vi "流程写入.vi"(11 "添加的路径":path) -> ()   [LabVIEW 2016, in "斯坦道总磷.lvlib"]
uses:
  <vilib>/Utility/miscctls.llb/LVPointTypeDef.ctl
panel:
  in  "关闭":bool
  out "字符串":string
  in  "加标回收":bool
  in  "标样核查":bool
  in  "跨度核查":bool
  in  "零点核查":bool
  in  "水样测量":bool=TRUE
  in  "写入":bool
  in  "参数下拉列表":enum16{"总磷", "总氮", "氨氮"}(ring)
  in  "量程下拉列表":enum16{"低量程", "高量程"}(ring)
  # "请选择要写入的流程"
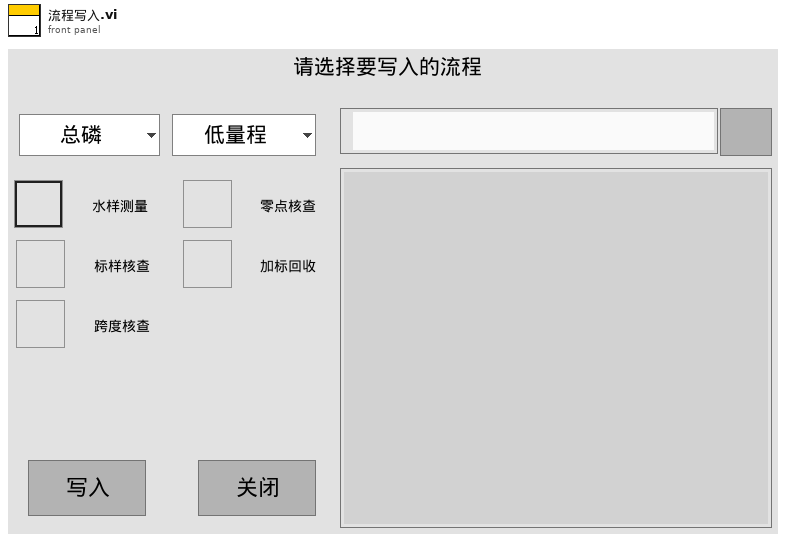
[diagram p1: front panel]
types:
  T1 = typedef "LVPointTypeDef.ctl" = cluster{"Horizontal":i16, "Vertical":i16}
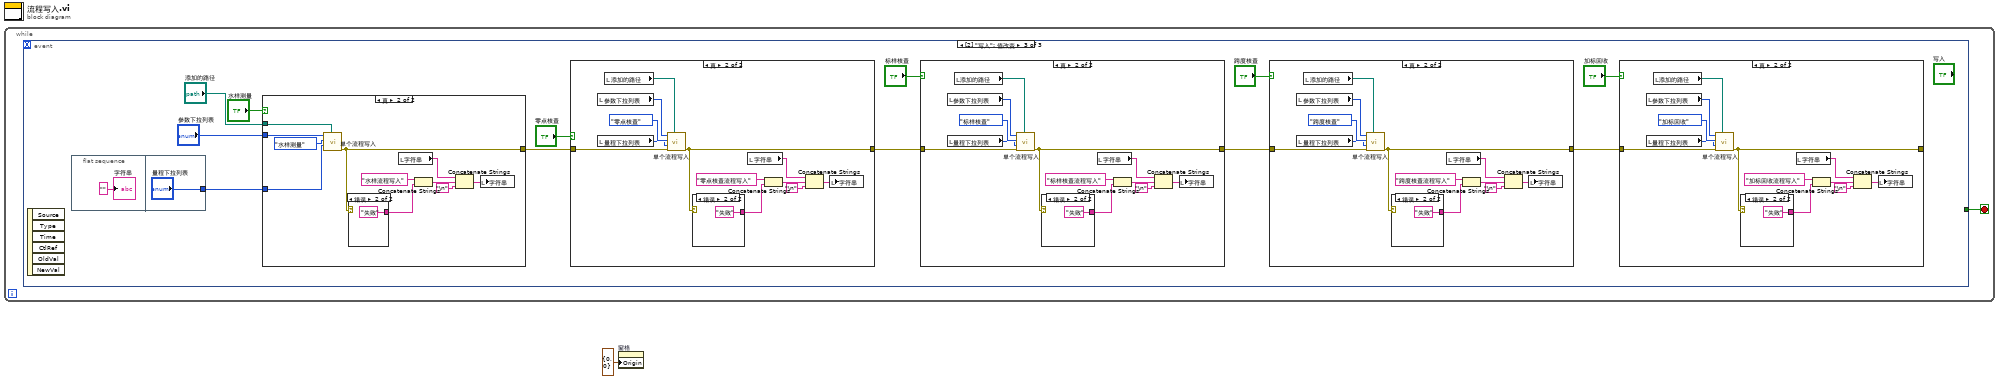
[diagram p0: block diagram]
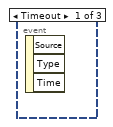
[diagram p2: hidden frame]
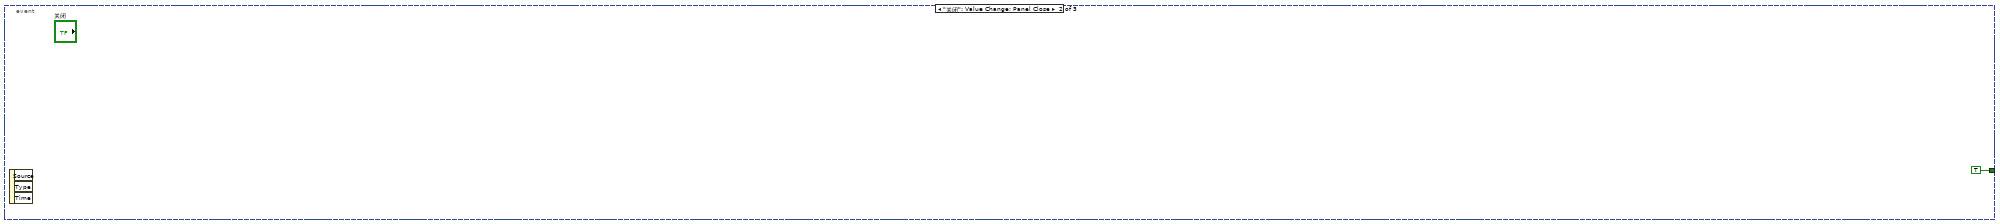
[diagram p3: hidden frame]
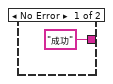
[diagram p5: hidden frame]
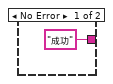
[diagram p7: hidden frame]
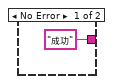
[diagram p9: hidden frame]
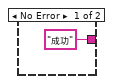
[diagram p11: hidden frame]
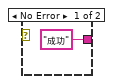
[diagram p13: hidden frame]
diagram:
  n1 = while {
    stop <- w2 stop-if-true
    n2 = event shown="[2] \"写入\": 值改变" {
      selector: _ -> [_ _ _]
      dyn-events: _ -> [_ _ _]
      timeout: _ -> [_ _ _]
      tunnel: [_ TRUE _] -> w2
      event Timeout {
        n3 = event-data() -> ()  [unwired: 1 in, 3 out]
      }
      event "关闭": Value Change; Panel Close {
        n4 = event-data() -> ()  [unwired: 1 in, 3 out]
      }
      event "写入": Value Change {
        n5 = event-data() -> ()  [unwired: 1 in, 6 out]
        n6 = flat-sequence {
          tunnel: ["量程下拉列表"] -> w14
          frame #0 {
            "字符串" <- ""
          }
          frame #1 {
          }
        }
        n7 = case shown="真" "水样测量" {
          tunnel: "添加的路径" -> [_ w84]
          tunnel: "参数下拉列表" -> [_ w83]
          tunnel: w14 -> [_ w82]
          tunnel: [_ w80] -> w11
          frame False {
          }
          frame True {
            n8 = call "单个流程写入.vi"("添加的路径"=w84, "量程"=w82, "测量模式"=enum16{"水样测量", "零点核查", "跨度核查", "标样核查", "加标回收"}."水样测量", "测量参数"=w83) -> ("error out"=w80:errorcluster)  [unwired: 7 in]
            n9 = case shown="错误" w80 {
              tunnel: ["成功" "失败"] -> w77
              frame No Error {
              }
              frame Error {
              }
            }
            n10 = local read "字符串"() -> (w79:string)
            n11 = Concatenate Strings("水样流程写入", w77) -> (w76:string)
            n12 = Concatenate Strings(w79, w76, "\n") -> (w74:string)
            n13 = local write "字符串"(w74) -> ()
          }
        }
        n14 = case shown="真" "零点核查" {
          tunnel: [_ w70] -> w9
          tunnel: w11 -> [_ w60]
          frame False {
          }
          frame True {
            n15 = local read "参数下拉列表"() -> (w62:enum16{"总磷", "总氮", "氨氮"})
            n16 = local read "量程下拉列表"() -> (w61:enum16{"低量程", "高量程"})
            n17 = local read "添加的路径"() -> (w63:path)
            n18 = call "单个流程写入.vi"("添加的路径"=w63, "error in (no error)"=w60, "量程"=w61, "测量模式"=enum16{"水样测量", "零点核查", "跨度核查", "标样核查", "加标回收"}."零点核查", "测量参数"=w62) -> ("error out"=w70:errorcluster)  [unwired: 6 in]
            n19 = case shown="错误" w70 {
              tunnel: ["成功" "失败"] -> w67
              frame No Error {
              }
              frame Error {
              }
            }
            n20 = local read "字符串"() -> (w69:string)
            n21 = Concatenate Strings("零点核查流程写入", w67) -> (w66:string)
            n22 = Concatenate Strings(w69, w66, "\n") -> (w64:string)
            n23 = local write "字符串"(w64) -> ()
          }
        }
        n24 = case shown="真" "标样核查" {
          tunnel: [_ w56] -> w7
          tunnel: w9 -> [_ w46]
          frame False {
          }
          frame True {
            n25 = local read "参数下拉列表"() -> (w48:enum16{"总磷", "总氮", "氨氮"})
            n26 = local read "量程下拉列表"() -> (w47:enum16{"低量程", "高量程"})
            n27 = local read "添加的路径"() -> (w49:path)
            n28 = call "单个流程写入.vi"("添加的路径"=w49, "error in (no error)"=w46, "量程"=w47, "测量模式"=enum16{"水样测量", "零点核查", "跨度核查", "标样核查", "加标回收"}."标样核查", "测量参数"=w48) -> ("error out"=w56:errorcluster)  [unwired: 6 in]
            n29 = case shown="错误" w56 {
              tunnel: ["成功" "失败"] -> w53
              frame No Error {
              }
              frame Error {
              }
            }
            n30 = local read "字符串"() -> (w55:string)
            n31 = Concatenate Strings("标样核查流程写入", w53) -> (w52:string)
            n32 = Concatenate Strings(w55, w52, "\n") -> (w50:string)
            n33 = local write "字符串"(w50) -> ()
          }
        }
        n34 = case shown="真" "跨度核查" {
          tunnel: [_ w32] -> w4
          tunnel: w7 -> [_ w33]
          frame False {
          }
          frame True {
            n35 = local read "参数下拉列表"() -> (w35:enum16{"总磷", "总氮", "氨氮"})
            n36 = local read "量程下拉列表"() -> (w34:enum16{"低量程", "高量程"})
            n37 = local read "添加的路径"() -> (w36:path)
            n38 = call "单个流程写入.vi"("添加的路径"=w36, "error in (no error)"=w33, "量程"=w34, "测量模式"=enum16{"水样测量", "零点核查", "跨度核查", "标样核查", "加标回收"}."跨度核查", "测量参数"=w35) -> ("error out"=w32:errorcluster)  [unwired: 6 in]
            n39 = case shown="错误" w32 {
              tunnel: ["成功" "失败"] -> w40
              frame No Error {
              }
              frame Error {
              }
            }
            n40 = local read "字符串"() -> (w42:string)
            n41 = Concatenate Strings("跨度核查流程写入", w40) -> (w39:string)
            n42 = Concatenate Strings(w42, w39, "\n") -> (w37:string)
            n43 = local write "字符串"(w37) -> ()
          }
        }
        n44 = case shown="真" "加标回收" {
          tunnel: [_ w28] -> _
          tunnel: w4 -> [_ w18]
          frame False {
          }
          frame True {
            n45 = local read "参数下拉列表"() -> (w20:enum16{"总磷", "总氮", "氨氮"})
            n46 = local read "量程下拉列表"() -> (w19:enum16{"低量程", "高量程"})
            n47 = local read "添加的路径"() -> (w21:path)
            n48 = call "单个流程写入.vi"("添加的路径"=w21, "error in (no error)"=w18, "量程"=w19, "测量模式"=enum16{"水样测量", "零点核查", "跨度核查", "标样核查", "加标回收"}."加标回收", "测量参数"=w20) -> ("error out"=w28:errorcluster)  [unwired: 6 in]
            n49 = case shown="错误" w28 {
              tunnel: ["成功" "失败"] -> w25
              frame No Error {
              }
              frame Error {
              }
            }
            n50 = local read "字符串"() -> (w27:string)
            n51 = Concatenate Strings("加标回收流程写入", w25) -> (w24:string)
            n52 = Concatenate Strings(w27, w24, "\n") -> (w22:string)
            n53 = local write "字符串"(w22) -> ()
          }
        }
      }
    }
  }
  n54 = property on="窗格" class="Pane"("Origin"=T1 {"Horizontal"=0, "Vertical"=0} ("原点")) -> ()  [unwired: 2 in, 2 out]
